vi "Z6_Beamline.PC Clear beamline.vi"(0 "i ref in":refnum<vi>, 5 "error IO":errorcluster) -> (14 "i ref out":refnum<vi>, 19 "error out":errorcluster)   [LabVIEW 2014, in "Z6_Beamline.lvlib"]
doc: "This is the Proc case \"Clear Beamline\"."
uses:
  Z6_Beamline.lvlib
  Z6_Beamline.Switch Instances.ctl
  Z6_Beamline.Black Box Instances.ctl
  PH_Switch/PH_Switch.lvlib
  PH_BL-Master/PH_BL-Master.lvlib
  PH_BlackBox/PH_BlackBox.lvlib
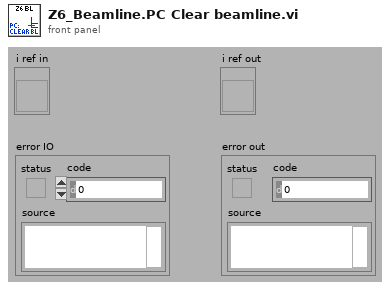
[diagram p1: front panel]
types:
  T1 = typedef "Z6_Beamline.lvlib/Z6_Beamline.Black Box Instances.ctl" = string
  T2 = typedef "Z6_Beamline.lvlib/Z6_Beamline.Switch Instances.ctl" = string
  T3 = typedef "Z6_Beamline.lvlib/Z6_Beamline.i attribute.ctl" = cluster{"Subs ok GUI Refs":T4, "Refs BL Northtower":refnum<vi>[], "Refs BL Southtower":refnum<vi>[], "Refs BL 100TW COS":refnum<vi>[], "State Subsystems":cluster{"Northtower":bool, "Southtower":bool, "Frontends":bool, "100TW COS":bool}, "Z6 Beamline Status Subscriber Information":T5, "Color State PHELIX":i16}
  T4 = typedef "Z6_Beamline.lvlib/Z6_Beamline.Subsystem ok GUI Refs.ctl" = cluster{"Northtower ok":refnum<vi>, "Southtower ok":refnum<vi>, "Frontends ok":refnum<vi>, "100TW COS ok":refnum<vi>}
  T5 = typedef "Z6_Beamline.lvlib/Z6_Beamline.Status Subscriber Information.ctl" = cluster{"BL Z6 Shutter":T6, "CH 10":T6, "CH 11":T6, "ST Flip Cam":T6, "ST Flip DB":T6, "BL Z6 Dump":T6}
  T6 = typedef "PH_BL-Master.lvlib/PH_BL-Master.Status Subscriber Information.ctl" = cluster{"Index of element":i32, "Attributeset":T7}
  T7 = typedef "PH_BL-Master.lvlib/PH_BL-Master.Attribute Set.ctl" = enum16{"Boolean Status Service Subscriber", "Picture Status Service Subscriber"}
  T8 = typedef "PH_StatusHandler.lvlib/PH_StatusHandler.Status.ctl" = i16
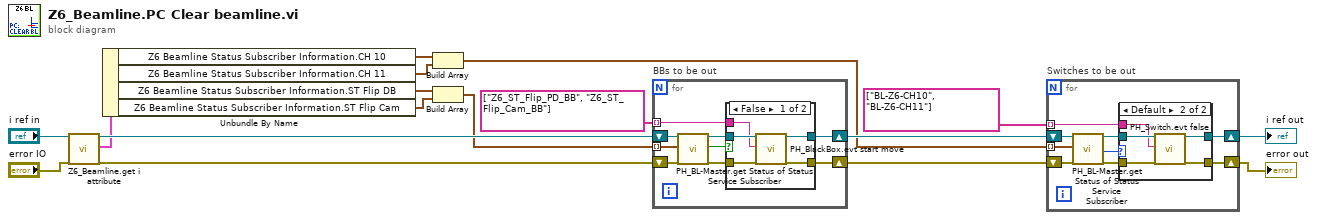
[diagram p0: block diagram]
diagram:
  n1 = call "Z6_Beamline.get i attribute.vi"("i ref in"="i ref in", "error in (no error)"="error IO") -> ("i ref out"=w9:refnum<vi>, "i attribute"=w8:T3, "error out"=w11:errorcluster)  [unwired: 15 in]
  n2 = Unbundle By Name(w8) -> ("Z6 Beamline Status Subscriber Information.CH 10"=w6:T6, "Z6 Beamline Status Subscriber Information.CH 11"=w5:T6, "Z6 Beamline Status Subscriber Information.ST Flip DB"=w7:T6, "Z6 Beamline Status Subscriber Information.ST Flip Cam"=w2:T6)
  n3 = Build Array(w6, w5) -> (w4:T6[])
  n4 = Build Array(w7, w2) -> (w3:T6[])
  n5 = for "BBs to be out" {
    tunnel: T1[] ["Z6_ST_Flip_PD_BB", "Z6_ST_Flip_Cam_BB"] -> [w22] mode=indexing
    tunnel: w3 -> [w18] mode=indexing
    shift-right: [w25] -> w13
    shift-left: w11 -> [w20]
    shift-right: [w23] -> w12
    shift-left: w9 -> [w19]
    n6 = call "PH_BL-Master.get Status of Status Service Subscriber.vi"("i ref in"=w19, "Wanted Status Subscriber Information"=w18, "error in (no error)"=w20) -> ("i ref out"=w24:refnum<vi>, "on/true/in?"=w21:bool, "error out"=w26:errorcluster)  [unwired: 11 in, 3 out]
    n7 = case shown="False" w21 {
      tunnel: w26 -> [w31 w32]
      tunnel: [w30 w32] -> w25
      tunnel: w24 -> [w29 w33]
      tunnel: [w28 w33] -> w23
      tunnel: w22 -> [w27 _]
      frame False {
        n8 = call "PH_BlackBox.evt start move.vi"("i ref in"=w29, "Instance"=w27, "error in (no error)"=w31) -> ("i ref out"=w28:refnum<vi>, "error out"=w30:errorcluster)  [unwired: 15 in]
      }
      frame True {
      }
    }
  }
  n9 = for "Switches to be out" {
    shift-right: [w39] -> w17
    shift-left: w13 -> [w42]
    shift-right: [w37] -> w16
    shift-left: w12 -> [w40]
    tunnel: T2[] ["BL-Z6-CH10", "BL-Z6-CH11"] -> [w35] mode=indexing
    tunnel: w4 -> [w34] mode=indexing
    n10 = call "PH_BL-Master.get Status of Status Service Subscriber.vi"("i ref in"=w40, "Wanted Status Subscriber Information"=w34, "error in (no error)"=w42) -> ("i ref out"=w38:refnum<vi>, "Status"=w36:T8, "error out"=w41:errorcluster)  [unwired: 11 in, 3 out]
    n11 = case shown="Default" w36 {
      tunnel: w41 -> [w43 w49]
      tunnel: [w43 w48] -> w39
      tunnel: w38 -> [w44 w47]
      tunnel: [w44 w46] -> w37
      tunnel: w35 -> [_ w45]
      frame 1 {
      }
      frame Default {
        n12 = call "PH_Switch.evt false.vi"("i ref in"=w47, "Instance"=w45, "error in (no error)"=w49) -> ("i ref out"=w46:refnum<vi>, "error out"=w48:errorcluster)  [unwired: 15 in]
      }
    }
  }
  "error out" <- w17
  "i ref out" <- w16
